vi "Example.vi"() -> ()   [LabVIEW 2026]
doc: "Uses a Web Browser to display web content."
panel:
  out "Web Browser Control":string(html)="http://localhost:5173/"
  in  "stop":bool
  out "WebData":string
  in  "URL String":string="http://localhost:5173/"
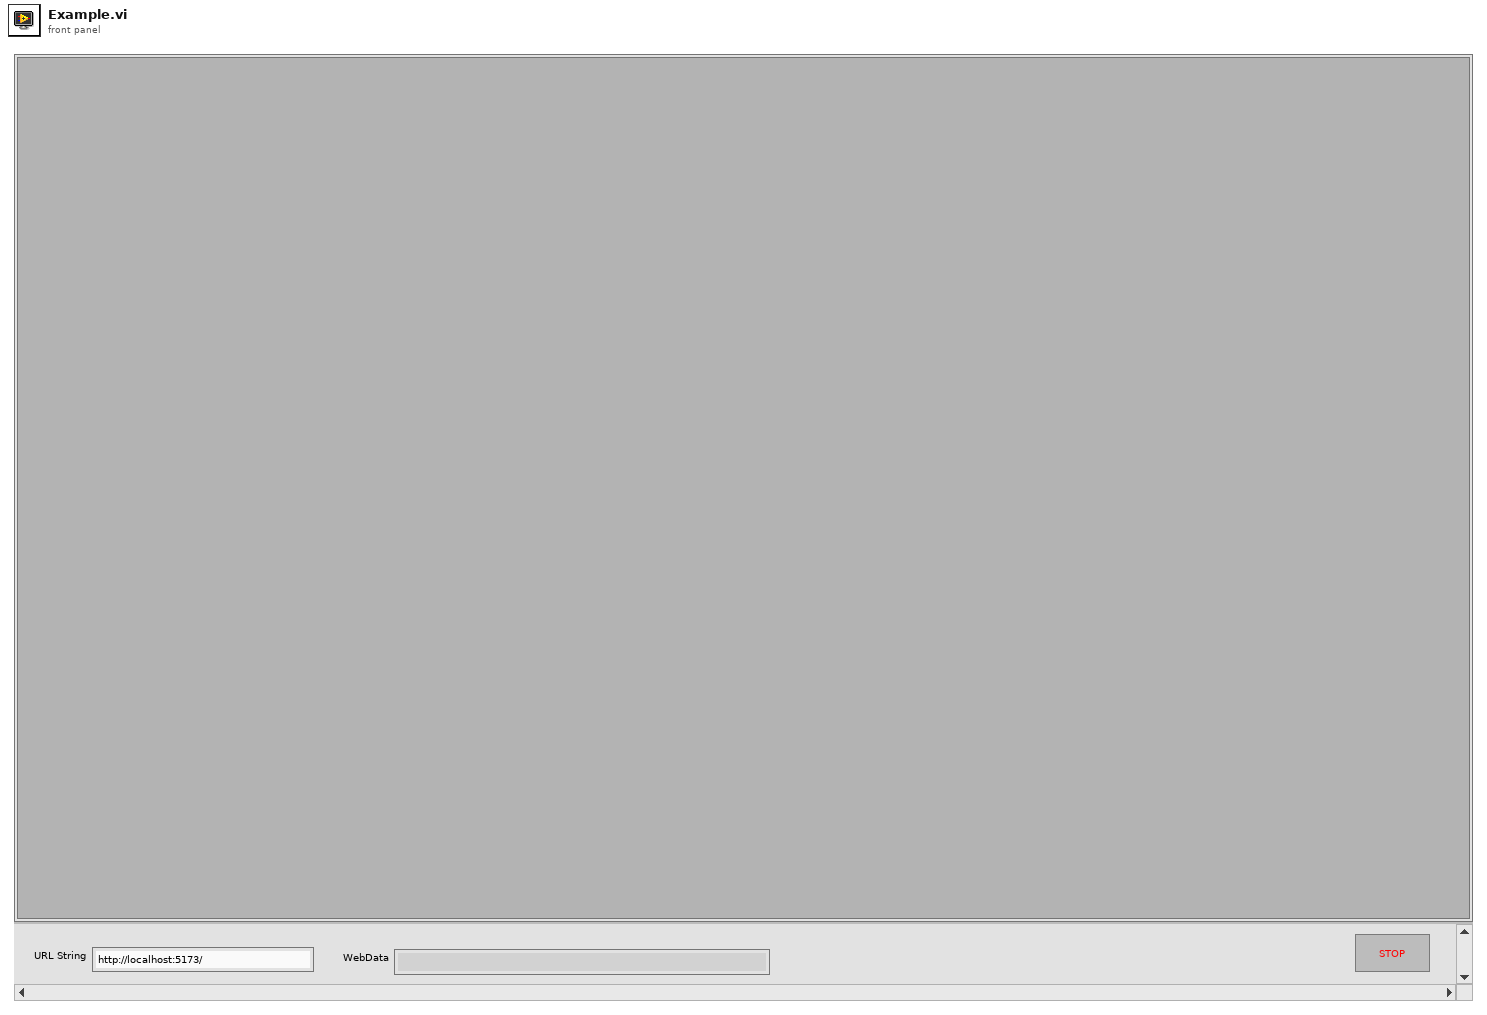
[diagram p1: front panel]
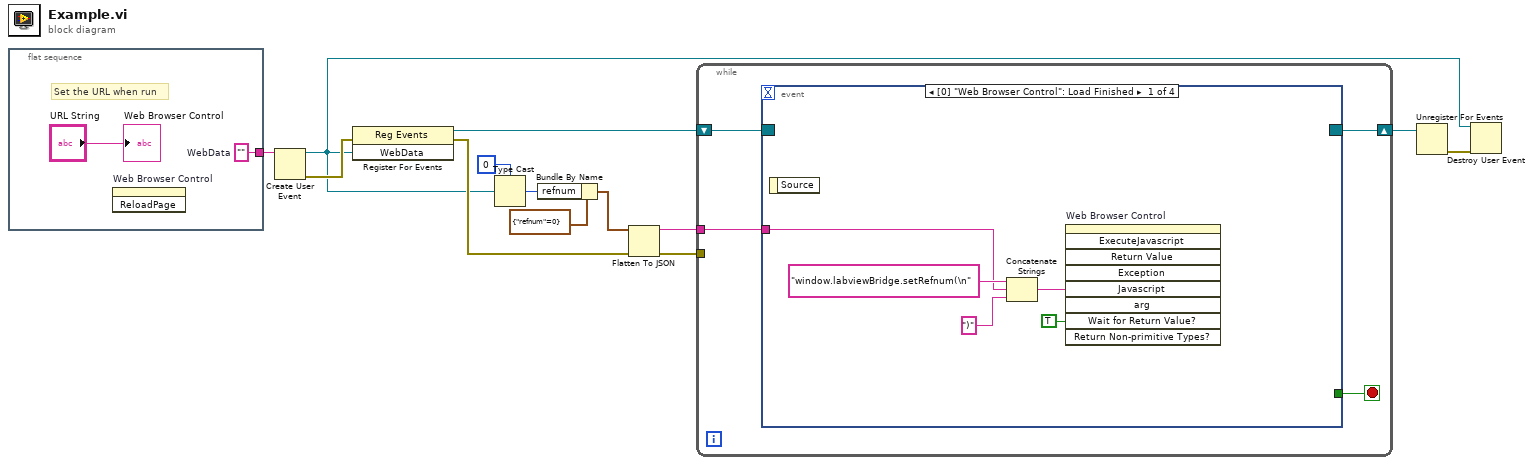
[diagram p0: block diagram]
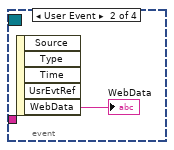
[diagram p2: hidden frame]
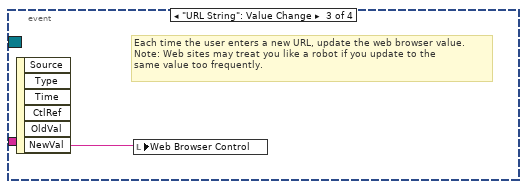
[diagram p3: hidden frame]
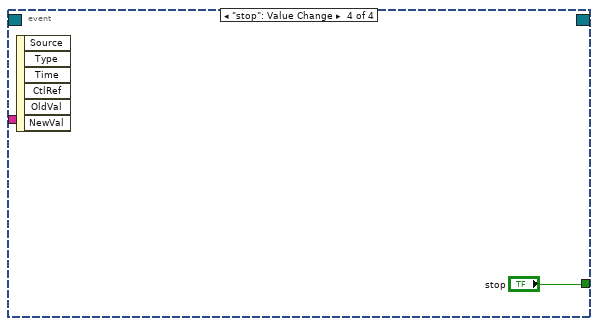
[diagram p4: hidden frame]
diagram:
  n1 = flat-sequence {
    tunnel: [w14] -> w1
    frame #0 {
      w14 = ""  # WebData
      # "Set the URL when run"
      n2 = invoke on="Web Browser Control" class="WebBrowser (strict)" method="ReloadPage"() -> ()  [unwired: 3 in, 3 out]
      "Web Browser Control" <- "URL String"
    }
  }
  n3 = Create User Event(user event datatype=w1) -> (user event=w2:refnum<user-event>, error out=w13:errorcluster)  [unwired: 1 in]
  n4 = register-events(error in=w13, w2) -> (reference out=w9:refnum<event-registration>, error out=w8:errorcluster)  [unwired: 1 in]
  n5 = Type Cast(type=u32 0, x=w2) -> (*(type *) &x=w4:u32)
  n6 = Bundle By Name(cluster=cluster{"refnum":u32} {"refnum"=0}, "refnum"=w4) -> (w11:cluster{"refnum":u32})
  n7 = Flatten To JSON(anything=w11, error in (no error)=w8) -> (JSON string=w3:string, 11:w7:errorcluster)  [unwired: 1 in]
  n8 = while {
    tunnel: w7 -> [_]
    tunnel: w3 -> [w16]
    shift-right: [w17] -> w5
    shift-left: w9 -> [w18]
    stop <- w19 stop-if-true
    n9 = event shown="[0] \"Web Browser Control\": Load Finished" {
      selector: w18 -> [_ _ _ _]
      dyn-events: [_ _ _ _] -> w17
      timeout: _ -> [_ _ _ _]
      tunnel: [_ _ _ "stop"] -> w19
      tunnel: w16 -> [w20 _ _ _]
      event "Web Browser Control": Load Finished {
        n10 = event-data() -> ()  [unwired: 1 in, 1 out]
        n11 = Concatenate Strings("window.labviewBridge.setRefnum(\n" ("Javascript String"), w20, ")" ("string")) -> (w22:string)
        n12 = invoke on="Web Browser Control" class="WebBrowser (strict)" method="ExecuteJavascript"("Javascript"=w22, "Wait for Return Value?"=TRUE) -> ()  [unwired: 7 in, 9 out]
      }
      event User Event {
        n13 = event-data() -> ("WebData"=→"WebData":string)  [unwired: 1 in, 4 out]
      }
      event "URL String": Value Change {
        # "Each time the user enters a new URL, update the web browser value.\nNote: Web sites may treat you like a robot if you update to the\nsame value too frequently."
        n14 = event-data() -> ("NewVal"=w26:string)  [unwired: 1 in, 5 out]
        n15 = local write "Web Browser Control"(w26) -> ()
      }
      event "stop": Value Change {
        n16 = event-data() -> ()  [unwired: 1 in, 6 out]
      }
    }
  }
  n17 = Unregister For Events(event registration refnum=w5) -> (error out=w6:errorcluster)  [unwired: 1 in]
  n18 = Destroy User Event(user event=w2, error in=w6) -> ()  [unwired: 1 out]
